vi "GetValueFromIndexes.vi"(1 "sweep_list":string[](array[string]), 2 "WorkFilePath":path, 3 "Sweep inst info":T1(array[cluster]), 4 "Indexes":u64[](array[numeric])) -> (0 "Points":cluster{"name":string, "data":u64, "data":dbl}[](array[cluster]))   [LabVIEW 2013]
uses:
  <vilib>/addons/h5labview2/base/lib_path.vi
  <vilib>/addons/h5labview2/base/H5Equery.vi
  <vilib>/addons/h5labview2/dataset/H5Dread.llb/H5Dread.xnode
  <vilib>/addons/h5labview2/base/hid_t.ctl
  <vilib>/addons/h5labview2/attrib/H5Aread.llb/H5Aread.xnode
  <vilib>/addons/h5labview2/dataset/H5D.lvlib
  <vilib>/addons/h5labview2/space/H5S.lvlib
  <vilib>/addons/h5labview2/file/H5F.lvlib
panel:
  out "elapsed time":u32
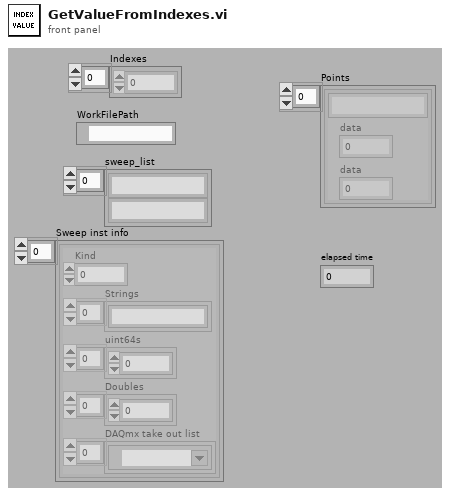
[diagram p1: front panel]
types:
  T1 = cluster{"Kind":u16, "Strings":string[], "uint64s":u64[], "Doubles":dbl[], "DAQmx take out list":refnum<k21>[]}[]
  T2 = typedef "hid_t.ctl" = i32
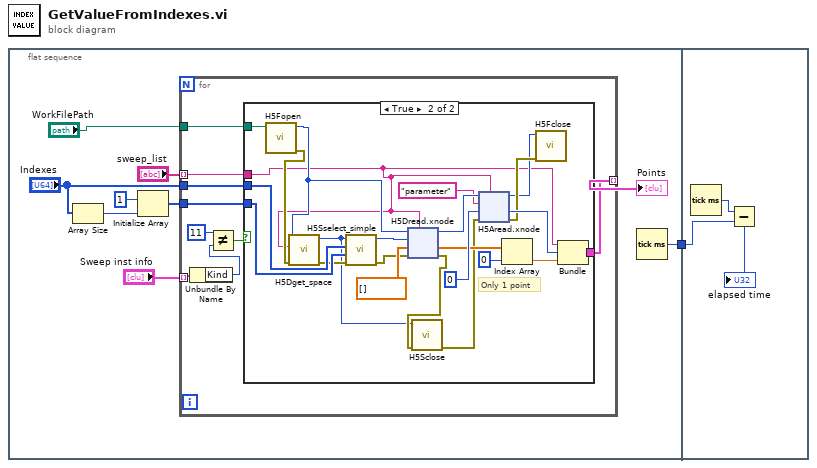
[diagram p0: block diagram]
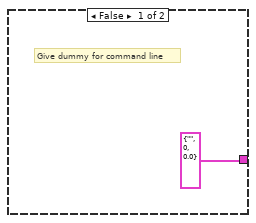
[diagram p2: hidden frame]
diagram:
  n1 = flat-sequence {
    tunnel: [w3] -> w1
    tunnel: w1 -> [w75]
    frame #0 {
      n2 = Array Size(array="Indexes") -> (size(s)=w9:i32)
      n3 = Initialize Array(u32 1, w9) -> (w5:u32[])
      n4 = for {
        tunnel: "sweep_list" -> [w16] mode=indexing
        tunnel: "Indexes" -> [w19]
        tunnel: w5 -> [w18]
        tunnel: [w17] -> w6 mode=indexing
        tunnel: "Sweep inst info" -> [w15] mode=indexing
        tunnel: "WorkFilePath" -> [w11]
        n5 = Unbundle By Name(w15) -> ("Kind"=w13:u16)
        n6 = Not Equal?(x=11, y=w13) -> (x != y?=w14:bool)
        n7 = case shown="True" w14 {
          tunnel: w19 -> [_ w43]
          tunnel: w18 -> [_ w42]
          tunnel: [cluster{"name":string, "data":u64, "data":dbl} {"name"="", "data"=0, "data"=0.0} w36] -> w17
          tunnel: w16 -> [_ w21]
          tunnel: w11 -> [_ w27]
          frame False {
            # "Give dummy for command line"
          }
          frame True {
            # "Only 1 point"
            n8 = call <vilib>:"H5Fopen.vi"("path"=w27) -> ("error out"=w26:errorcluster, "ref out"=w25:T2)  [unwired: 9 in]
            n9 = call <vilib>:"H5Dget_space.vi"("error in (no error)"=w26, "obj (.)"=w21, "ref in"=w25) -> ("error out"=w31:errorcluster, "space out"=w28:T2)  [unwired: 7 in]
            n10 = call <vilib>:"H5Sselect_simple.vi"("error in (no error)"=w31, "count"=w42, "start"=w43, "space in"=w28) -> ("error out"=w30:errorcluster, "space out"=w41:T2)  [unwired: 6 in]
            n11 = xnode "H5Dread.xnode"("dataset name (this)"=w21, "error in (no error)"=w30, "default"=dbl[] [], "file space"=w41, "ref in"=w25) -> ("error out"=w29:errorcluster, "data"=w34:dbl[], "ref out"=w40:T2)  [unwired: 1 in, 1 out]
            n12 = call <vilib>:"H5Sclose.vi"("error in (no error)"=w29, "space in"=w28) -> ("error out"=w24:errorcluster)  [unwired: 9 in]
            n13 = xnode "H5Aread.xnode"("object name"=w21, "error in (no error)"=w24, "default"=u16 0, "attrib name"="parameter", "ref in"=w40) -> ("error out"=w23:errorcluster, "data"=w37:u16, "ref out"=w22:T2)  [unwired: 1 in, 1 out]
            n14 = Index Array(array=w34, index=0) -> (element=w33:dbl)
            n15 = call <vilib>:"H5Fclose.vi"("error in (no error)"=w23, "ref"=w22) -> ()  [unwired: 9 in, 1 out]
            n16 = Bundle(w21, "data"=w37, w33) -> (w36:cluster{string, "data":u16, dbl})  [unwired: 1 in]
          }
        }
      }
      "Points" <- w6
      n17 = Tick Count (ms)() -> (millisecond timer value=w3:u32)
    }
    frame #1 {
      n18 = Tick Count (ms)() -> (millisecond timer value=w76:u32)
      n19 = Subtract(x=w76, y=w75) -> (x-y=→"elapsed time":u32)
    }
  }
